vi "Handle Error.vi"(8 "error in (no error)":errorcluster, 11 "WebSocket Server Manager in":refnum<class "WebSocket Server Manager.lvclass">) -> (0 "error out":errorcluster, 2 "stop actor?":bool=TRUE, 3 "WebSocket Server Manager out":refnum<class "WebSocket Server Manager.lvclass">)   [LabVIEW 2021, in "WebSocket Actors.lvlib" / "WebSocket Server Manager.lvclass"]
doc: "(<B>Filename</B>: Actor Framework.lvlib:Actor.lvclass:Handle Error.vi)\n\nDefines how the actor handles an error that occurred while processing a message. By default, this method does nothing except stop the actor."
uses:
  WebSocket Server Manager.lvclass
  C:/Program Files/National Instruments/LabVIEW 2021/vi.lib/ActorFramework/Actor/Actor.lvclass
  <vilib>/ActorFramework/Actor/Actor.lvclass/Actor.ctl
  <vilib>/ActorFramework/Report Error Msg/Report Error Msg.lvclass/Report Error Msg.ctl
  <vilib>/ActorFramework/Message Enqueuer/Message Enqueuer.lvclass/Message Enqueuer.ctl
  <vilib>/ActorFramework/Message Enqueuer/Enqueue.vi
  <vilib>/ActorFramework/Report Error Msg/Report Error Msg.lvclass
  C:/Program Files/National Instruments/LabVIEW 2021/vi.lib/ActorFramework/Message/Message.lvclass
  <vilib>/Utility/LVClass/Get LV Class Name.vi
  <resource>/AFDebug/Generate Trace for Message.vi
  <vilib>/ActorFramework/Message Priority Queue/Priority Enqueue.vi
  WebSocket Server Manager.lvclass/WebSocket Server Manager.ctl
  <vilib>/ActorFramework/Actor/Actor.lvclass
  <userlib>/_OpenG.lib/error/error.llb/openg_error.lvlib
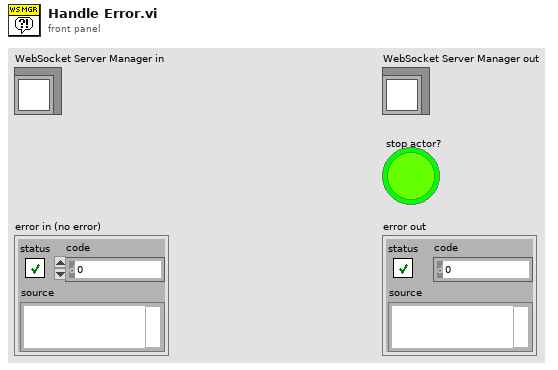
[diagram p1: front panel]
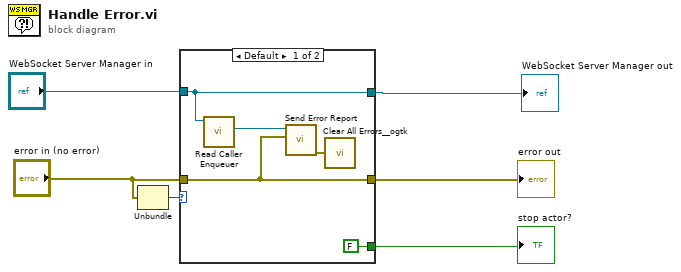
[diagram p0: block diagram]
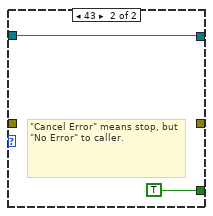
[diagram p2: hidden frame]
diagram:
  n1 = Unbundle("error in (no error)") -> ("code"=w6:i32)  [unwired: 2 out]
  n2 = case shown="Default" w6 {
    tunnel: [w10 _] -> w4
    tunnel: "error in (no error)" -> [w10 _]
    tunnel: [FALSE ("stop actor?") TRUE ("stop actor?")] -> w3
    tunnel: "WebSocket Server Manager in" -> [w8 w12]
    tunnel: [w8 w12] -> w2
    frame Default {
      n3 = call <vilib>:"Read Caller Enqueuer.vi"("Actor"=w8) -> ("Caller Enqueuer"=w11:refnum<class "Message Enqueuer.lvclass">)  [unwired: 10 in]
      n4 = call <vilib>:"Send Error Report.vi"("Error From Sender"=w10, "Message Enqueuer"=w11) -> ("error out"=w7:errorcluster)  [unwired: 9 in]
      n5 = call <userlib>:"Clear All Errors__ogtk.vi"("Error In"=w7) -> ()  [unwired: 3 in, 1 out]
    }
    frame 43 {
      # "\"Cancel Error\" means stop, but \"No Error\" to caller."
    }
  }
  "WebSocket Server Manager out" <- w2
  "error out" <- w4
  "stop actor?" <- w3
